vi "AlazarGetWhotriggeredBySystemID.vi"(3 "error in (no error)":errorcluster, 4 "Record Number":u32, 5 "Board ID":u32, 6 "System ID":u32) -> (0 "error out":errorcluster, 2 "Who":u32(ring) items=["Not this board", "Channel A", "Channel B", "Ext. Trig. In", "Ch. A and ch. B", "Ch. A and Ext. Trig. In.", "Ch. B and Ext. Trig. In.", "Trigger Timeout"])   [LabVIEW 2018]
doc: "Return which event caused a board system to trigger and capture a record to on-board memory."
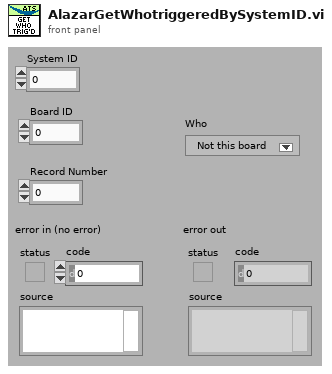
[diagram p1: front panel]
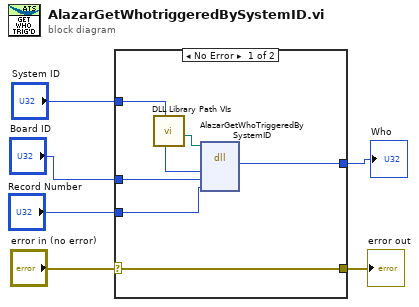
[diagram p0: block diagram]
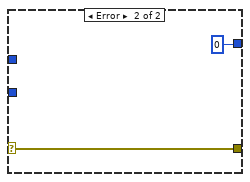
[diagram p2: hidden frame]
diagram:
  n1 = case shown="No Error" "error in (no error)" {
    selector: "error in (no error)" -> [w11 w14]
    tunnel: [w11 w14] -> w5
    tunnel: "System ID" -> [w12 _]
    tunnel: "Board ID" -> [w10 _]
    tunnel: "Record Number" -> [w9 _]
    tunnel: [w8 u32 0] -> w1
    frame No Error {
      n2 = call "DLL Library Path VIs.vi"() -> ("Alazar"=w7:path)  [unwired: 9 in, 2 out]
      n3 = dll-call lib="C:/Project/SerialSectOCT - FFT GPU/SerialSectOCT/Labview Software/DLL/ATSApi.dll" fn="AlazarGetWhoTriggeredBySystemID"(path in=w7, "systemId"=w12, "boardID"=w10, "recordNumber"=w9) -> ("return type"=w8:u32)  [unwired: 5 in, 2 out]
    }
    frame Error {
    }
  }
  "error out" <- w5
  "Who" <- w1
